vi "rvc Skew-Symmetric Matrix to Vector.vi"(11 "output variable in":dbl[][](array[numeric])) -> (3 "output variable out":dbl[](array[numeric]))   [LabVIEW 2013]
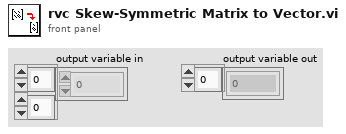
[diagram p1: front panel]
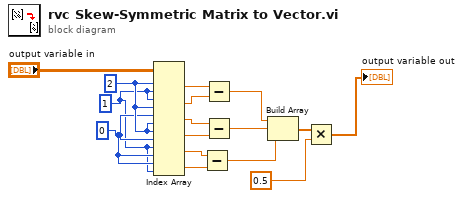
[diagram p0: block diagram]
diagram:
  w10 = 0 ("disabled index (col)")
  w9 = 1 ("disabled index (col)")
  w11 = 2 ("index (row)")
  n1 = Index Array(array="output variable in", index (row) #1=w11, index (col) #1=w9, index (row) #2=w9, index (col) #2=w11, index (row) #3=w10, index (col) #3=w11, index (row) #4=w11, index (col) #4=w10, index (row) #5=w9, index (col) #5=w10, index (row) #6=w10, index (col) #6=w9) -> (element #1=w14:dbl, element #2=w15:dbl, element #3=w12:dbl, element #4=w13:dbl, element #5=w7:dbl, element #6=w8:dbl)
  n2 = Subtract(x=w7, y=w8) -> (x-y=w4:dbl)
  n3 = Subtract(x=w14, y=w15) -> (x-y=w6:dbl)
  n4 = Subtract(x=w12, y=w13) -> (x-y=w5:dbl)
  n5 = Build Array(w6, w5, w4) -> (w3:dbl[])
  n6 = Multiply(x=w3, y=0.5 ("x-y")) -> (x*y=→"output variable out":dbl[])
